vi "Read SSH.vi"(8 "Error In":errorcluster, 11 "SFTP Directory In":refnum<class "SFTP Directory.lvclass">) -> (0 "Error Out":errorcluster, 2 "SSH":refnum<class "SSH.lvclass">, 3 "SFTP Directory Out":refnum<class "SFTP Directory.lvclass">)   [LabVIEW 2018, in "Toolkit.lvlib" / "SFTP Directory.lvclass"]
doc: "Gets the SSH context used to create this SFTP Directory object."
uses:
  SFTP Directory.lvclass
  SSH/SSH.lvclass
  SFTP Directory.lvclass/SFTP Directory.ctl
  SFTP/SFTP.lvclass/SFTP.ctl
  Session/Session.lvclass/Session.ctl
  SFTP/SFTP.lvclass
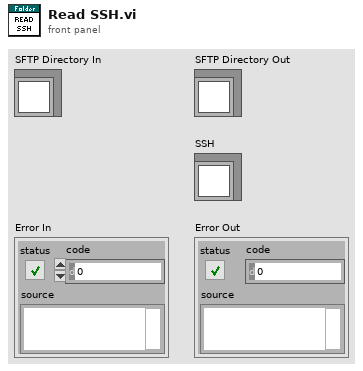
[diagram p1: front panel]
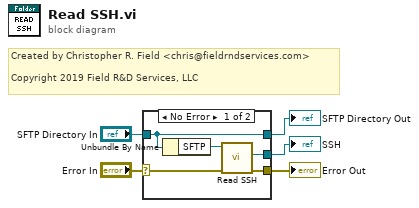
[diagram p0: block diagram]
diagram:
  # "Created by Christopher R. Field <chris@fieldrndservices.com>\n\nCopyright 2019 Field R&D Services, LLC"
  n1 = case shown="No Error" "Error In" {
    selector: "Error In" -> [w7 w12]
    tunnel: "SFTP Directory In" -> [w10 w11]
    tunnel: [w10 w11] -> w3
    tunnel: [w6 w12] -> w2
    tunnel: [w8 _] -> w1
    frame No Error {
      n2 = Unbundle By Name(w10) -> ("SFTP"=w9:refnum<class "SFTP.lvclass">)
      n3 = call "Read SSH.vi"("Error In"=w7, "SFTP In"=w9) -> ("Erorr Out"=w6:errorcluster, "SSH"=w8:refnum<class "SSH.lvclass">)  [unwired: 7 in, 1 out]
    }
    frame Error {
    }
  }
  "SFTP Directory Out" <- w3
  "Error Out" <- w2
  "SSH" <- w1
